vi "derivative.vi"(8 "step_size":dbl, 9 "gain":dbl=1.0, 10 "input":dbl) -> (2 "output":dbl)   [LabVIEW 2015]
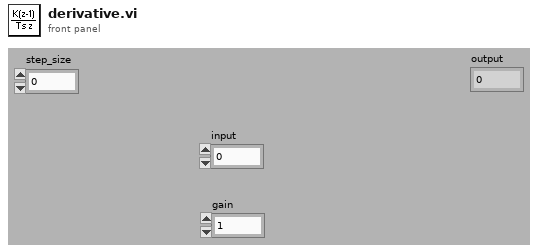
[diagram p1: front panel]
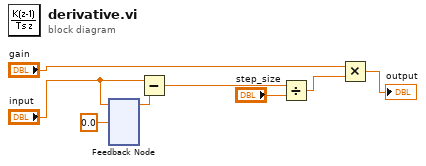
[diagram p0: block diagram]
diagram:
  n1 = feedback-in #1("input") -> ()
  n2 = feedback #1(0.0 ("input")) -> (w5:dbl)
  n3 = Subtract(x="input", y=w5) -> (x-y=w6:dbl)
  n4 = Divide(x=w6, y="step_size") -> (x/y=w7:dbl)
  n5 = Multiply(x="gain", y=w7) -> (x*y=→"output":dbl)
